vi "openFile.vi"(8 "error in (no error)":errorcluster, 10 "path":path) -> (0 "error out":errorcluster, 2 "Refnum Cluster Out":T1)   [LabVIEW 2012]
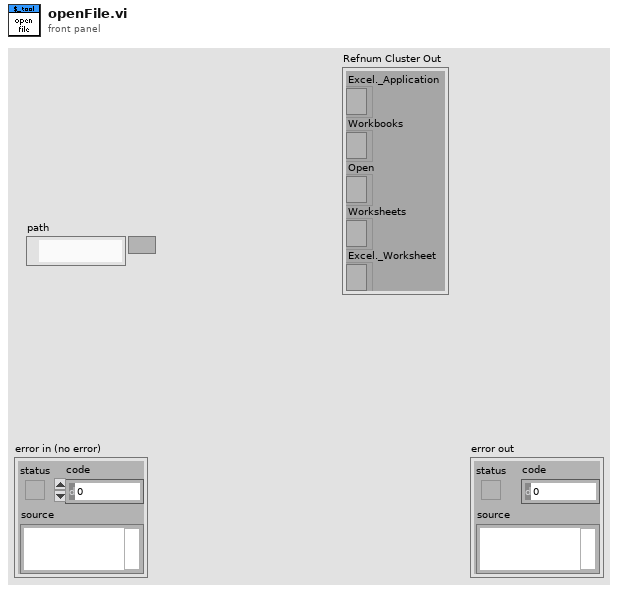
[diagram p1: front panel]
types:
  T1 = cluster{"Excel._Application":refnum<k7>, "Workbooks":refnum<k7>, "Open":refnum<k7>, "Worksheets":refnum<k7>, "Excel._Worksheet":refnum<k7>}
  T2 = cluster{"Excel._Application":refnum<k7>, "Workbooks":refnum<k7>}
  T3 = cluster{"Excel._Application":refnum<k7>, "Workbooks":refnum<k7>, "Open":refnum<k7>}
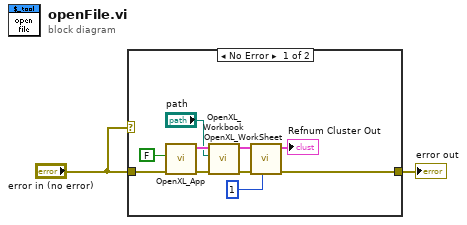
[diagram p0: block diagram]
diagram:
  n1 = case shown="No Error" "error in (no error)" {
    tunnel: "error in (no error)" -> [w5 w13]
    tunnel: [w4 w13] -> w2
    frame No Error {
      n2 = call <userlib>:"OpenXL_App.vi"("error in (no error)"=w5, "Visible"=FALSE) -> ("error out"=w10:errorcluster, "Refnum Cluster"=w11:T2)  [unwired: 8 in]
      n3 = call <userlib>:"OpenXL_Workbook.vi"("error in"=w10, "path"="path", "Refnum Cluster In"=w11) -> ("error out"=w8:errorcluster, "Refnum Cluster Out"=w9:T3)  [unwired: 7 in]
      n4 = call <userlib>:"OpenXL_WorkSheet.vi"("Sheet"=1, "error in (no error)"=w8, "Refnum Cluster In"=w9) -> ("error out"=w4:errorcluster, "Refnum Cluster Out"=→"Refnum Cluster Out":T1)  [unwired: 7 in]
    }
    frame Error {
    }
  }
  "error out" <- w2
